vi "Set Data.vi"(8 "error in (no error)":errorcluster, 9 "Offset":i32, 10 "Data in":string, 11 "Content in":T1) -> (0 "error out":errorcluster, 3 "Content out":T1)   [LabVIEW 2021, in "VI-Hacker.lvlib"]
uses:
  VI-Hacker.lvlib
  TypeDefs/Content.ctl
  TypeDefs/Block.ctl
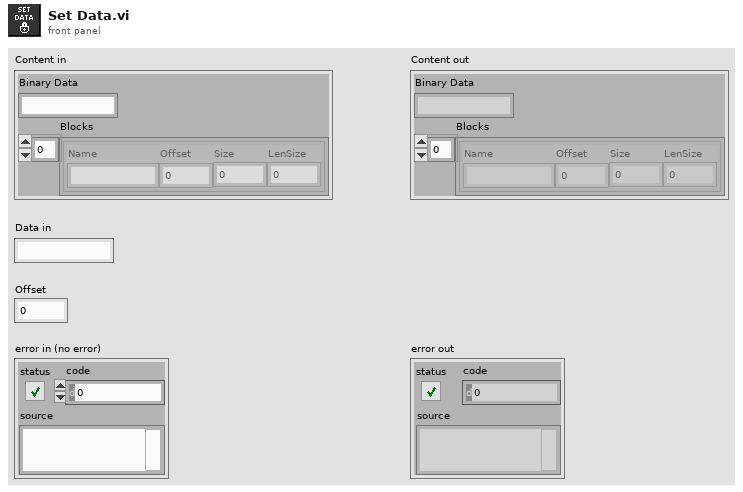
[diagram p1: front panel]
types:
  T1 = typedef "VI-Hacker.lvlib/Content.ctl" = cluster{"Binary Data":string, "Blocks":T2[]}
  T2 = typedef "VI-Hacker.lvlib/Block.ctl" = cluster{"Name":string, "Offset":i32, "Size":i32, "LenSize":i32}
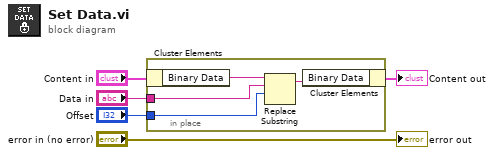
[diagram p0: block diagram]
diagram:
  n1 = in-place {
    in-place-border: "Data in" -> [w7]
    in-place-border: "Offset" -> [w6]
    n2 = in-place-cluster #1("Content in") -> ("Binary Data"=w9:string)
    n3 = Replace Substring(3:w6, 4:w7, 5:w9) -> (1:w8:string)  [unwired: 1 in, 1 out]
    n4 = in-place-cluster #1("Binary Data"=w8) -> (→"Content out":T1)
  }
  "error out" <- "error in (no error)"
